vi "MauiTemplate.TestLauncher.vi"() -> ()   [LabVIEW 2016, in "MauiTemplate.lvclass"]
uses:
  MauiTemplate.lvclass
  <vilib>/JKI/JKI SMO/SMO/Typedefs/SMOState --Enum.ctl
  C:/Program Files (x86)/National Instruments/LabVIEW 2016/vi.lib/JKI/JKI SMO/SMO/SMO.lvclass
  C:/Program Files (x86)/National Instruments/LabVIEW 2016/vi.lib/JKI/JKI SMO/SMO.UI/SMO.UI.lvclass
  <vilib>/JKI/JKI SMO/SMO/SMO.lvclass
  <vilib>/JKI/JKI SMO/SMO.UI/SMO.UI.lvclass
panel:
  out "SMO State":T1
  out "error out":errorcluster
  in  "Stop":bool
  # "Basic SMO Test Launcher"
  # "For instructions on how to use the JKI State Machine Objects, examples and video tutorials, visit:\nhttp://jki.net/state-machine-objects/\n\nJKI State Machine Objects™\nhttp://jki.net/state-machine-objects/\nCopyright (C) 2005-2015, JKI <info@jki.net>\nALL RIGHTS RESERVED"
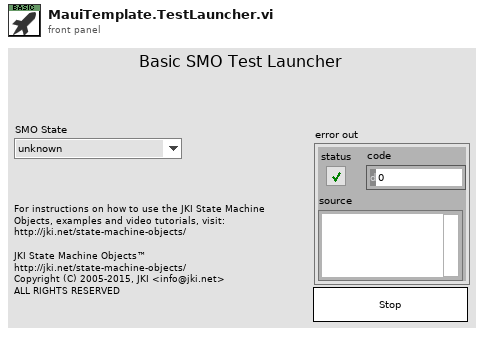
[diagram p1: front panel]
types:
  T1 = typedef "SMO.lvclass/SMOState --Enum.ctl" = enum16{"unknown", "Created", "Started", "Stopped"}
  T2 = typedef "SMO.lvclass/Public Events.ctl" = cluster{"Error":refnum<user-event>, "State":refnum<user-event>, "Reserve State":refnum<user-event>}
  T3 = typedef "SMO.UI.lvclass/PublicEvents--Cluster.ctl" = cluster{"UI Hidden":refnum<user-event>, "UI State":refnum<user-event>}
  T4 = cluster{"Event Registration Refnum":refnum<event-registration>}
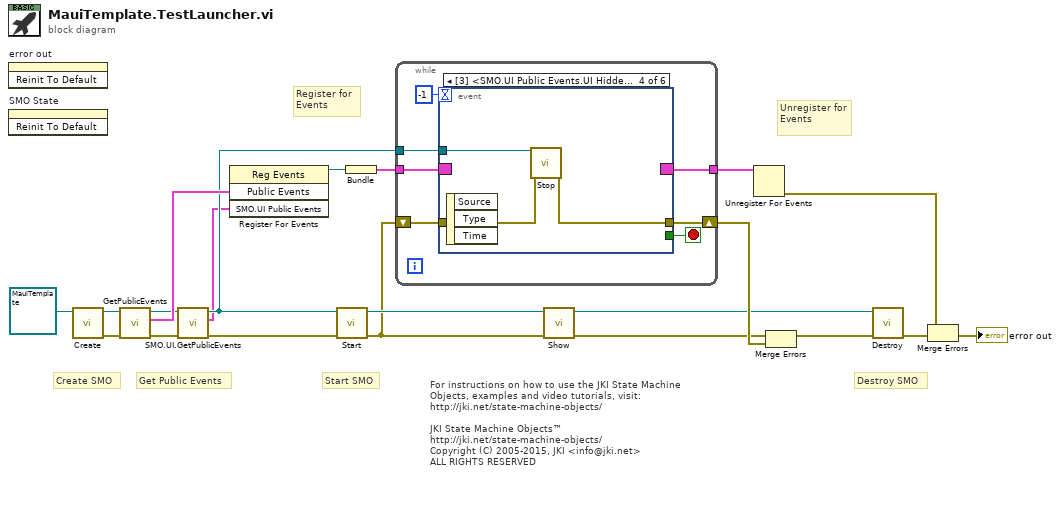
[diagram p0: block diagram]
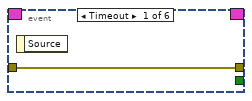
[diagram p2: hidden frame]
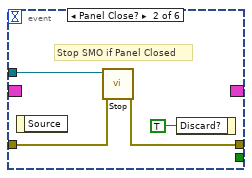
[diagram p3: hidden frame]
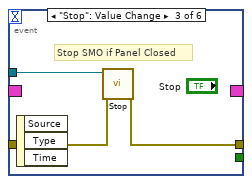
[diagram p4: hidden frame]
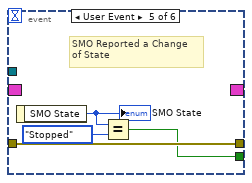
[diagram p5: hidden frame]
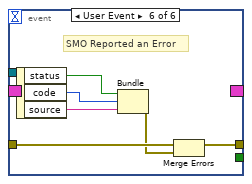
[diagram p6: hidden frame]
diagram:
  # "For instructions on how to use the JKI State Machine Objects, examples and video tutorials, visit:\nhttp://jki.net/state-machine-objects/\n\nJKI State Machine Objects™\nhttp://jki.net/state-machine-objects/\nCopyright (C) 2005-2015, JKI <info@jki.net>\nALL RIGHTS RESERVED"
  # "Get Public Events"
  # "Start SMO"
  # "Destroy SMO"
  # "Create SMO"
  # "Unregister for Events"
  # "Register for Events"
  n1 = invoke on="error out" class="Clust (strict)" method="Reinit To Default"() -> ()  [unwired: 3 in, 3 out]
  n2 = invoke on="SMO State" class="Enum (strict)" method="Reinit To Default"() -> ()  [unwired: 3 in, 3 out]
  n3 = call <vilib>:"Create.vi"("SMO"=refnum<class "MauiTemplate.lvclass"> refnum ("SMO.Template.lvclass")) -> ("error out"=w11:errorcluster, "SMO out"=w12:refnum<class "MauiTemplate.lvclass">)  [unwired: 8 in, 1 out]
  n4 = call <vilib>:"GetPublicEvents.vi"("error in (no error)"=w11, "SMO"=w12) -> ("error out"=w10:errorcluster, "Public Events"=w9:T2, "SMO out"=w3:refnum<class "MauiTemplate.lvclass">)  [unwired: 7 in]
  n5 = call <vilib>:"SMO.UI.GetPublicEvents.vi"("SMO.UI"=w3) -> ("SMO.UI Public Events"=w1:T3, "SMO.UI out"=w2:refnum<class "MauiTemplate.lvclass">)  [unwired: 8 in, 1 out]
  n6 = register-events(w9, w1) -> (reference out=w8:refnum<event-registration>)  [unwired: 2 in, 1 out]
  n7 = call <vilib>:"Start.vi"("error in (no error)"=w10, "SMO"=w2) -> ("error out"=w5:errorcluster, "SMO out"=w7:refnum<class "MauiTemplate.lvclass">)  [unwired: 8 in]
  n8 = Bundle("Event Registration Refnum"=w8) -> (w19:T4)  [unwired: 1 in]
  n9 = while {
    shift-right: [w26] -> w18
    shift-left: w5 -> [w25]
    tunnel: w19 -> [w24]
    tunnel: [w23] -> w20
    tunnel: w2 -> [w22]
    stop <- w27 stop-if-true
    n10 = event shown="[3] <SMO.UI Public Events.UI Hidden>: User Event" {
      selector: w24 -> [_ _ _ _ _ _]
      dyn-events: [_ _ _ _ _ _] -> w23
      timeout: -1 -> [_ _ _ _ _ _]
      tunnel: [_ _ _ _ w39 _] -> w27
      tunnel: w22 -> [_ w32 w35 w38 _ _]
      tunnel: [w28 w31 w34 w36 w42 w46] -> w26
      tunnel: w25 -> [w28 w30 w33 w37 w42 w44]
      event Timeout {
        n11 = event-data() -> ()  [unwired: 1 in, 1 out]
      }
      event Panel Close? {
        # "Stop SMO if Panel Closed"
        n12 = event-data() -> ()  [unwired: 1 in, 1 out]
        n13 = call <vilib>:"Stop.vi"("error in (no error)"=w30, "SMO"=w32) -> ("error out"=w31:errorcluster)  [unwired: 8 in, 1 out]
        n14 = event-data("Discard?"=TRUE ("OK")) -> ()  [unwired: 1 in, 1 out]
      }
      event "Stop": Value Change {
        # "Stop SMO if Panel Closed"
        n15 = event-data() -> ()  [unwired: 1 in, 3 out]
        n16 = call <vilib>:"Stop.vi"("error in (no error)"=w33, "SMO"=w35) -> ("error out"=w34:errorcluster)  [unwired: 8 in, 1 out]
      }
      event User Event {
        n17 = event-data() -> ()  [unwired: 1 in, 3 out]
        n18 = call <vilib>:"Stop.vi"("error in (no error)"=w37, "SMO"=w38) -> ("error out"=w36:errorcluster)  [unwired: 8 in, 1 out]
      }
      event User Event {
        # "SMO Reported a Change\nof State"
        n19 = event-data() -> ("SMO State"=w41:T1)  [unwired: 1 in]
        "SMO State" <- w41
        n20 = Equal?(x=w41, y=SMOState_--Enum."Stopped") -> (x = y?=w39:bool)
      }
      event User Event {
        # "SMO Reported an Error"
        n21 = event-data() -> ("status"=w45:bool, "code"=w48:i32, "source"=w47:string)  [unwired: 1 in]
        n22 = Bundle("status"=w45, "code"=w48, "source"=w47) -> (w43:errorcluster)  [unwired: 1 in]
        n23 = Merge Errors(w44, w43) -> (w46:errorcluster)
      }
    }
  }
  n24 = call <vilib>:"Show.vi"("error in (no error)"=w5, "SMO.UI"=w7) -> ("error out"=w4:errorcluster, "SMO.UI out"=w6:refnum<class "MauiTemplate.lvclass">)  [unwired: 8 in]
  n25 = Unregister For Events(event registration refnum=w20) -> (error out=w17:errorcluster)  [unwired: 1 in]
  n26 = Merge Errors(w4, w18) -> (w13:errorcluster)
  n27 = call <vilib>:"Destroy.vi"("error in (no error)"=w13, "SMO"=w6) -> ("error out"=w15:errorcluster)  [unwired: 9 in]
  n28 = Merge Errors(w17, w15) -> (→"error out":errorcluster)
